vi "SQL模块化.vi"(0 "Database name":string="Test_Database", 1 "Table name":string="Test_Database", 2 "operate option":T1(ring)=enum."Select Data", 3 "primary key (-1)":i32=-1, 4 "Column information":T2[](array[typedef])=[{"column name"="ID", "data type"=enum."Long (I32)", "size"=50, "allow null?"=FALSE}, {"column name"="name", "data type"=enum."String", "size"=50, "allow null?"=TRUE}, {"column name"="number", "data type"=enum."Long (I32)", "size"=50, "allow null?"=TRUE}, {"column name"="date", "data type"=enum."Date/Time", "size"=50, "allow null?"=TRUE}], 5 "Column name":string="ID", 6 "Additional":string, 7 "error in (no error)":errorcluster, 9 "Update Column name":string="name", 10 "Insert Data":string[](array[string])=["5", "D", "5", "2015/1/19 14:41:15"], 11 "Update Data":string="E", 12 "Delete Search Condition":string="ID", 13 "Update Search Condition":string="ID", 14 "Delete Search Condition Value":string="5", 15 "Update Search Condition Value":string="5") -> (8 "columns":string[](array[string])=["ID", "name", "number", "date"], 20 "Data Out":string[][](array[string]), 27 "error out":errorcluster)   [LabVIEW 2017]
uses:
  <vilib>/addons/database/Auxilliary.llb/DB Tools Column Info.ctl
  <vilib>/addons/database/Auxilliary.llb/DB Tools DataTypes.ctl
  <vilib>/addons/database/Auxilliary.llb/DB Tools Transaction.ctl
  <vilib>/addons/database/Connection.llb/DB Tools Open Connec (String).vi
  <vilib>/addons/database/Connection.llb/Conn Transaction.vi
  <vilib>/addons/database/Connection.llb/Conn Execute.vi
  <vilib>/addons/database/Recordset.llb/Rec Fetch Recordset Data (R).vi
  <vilib>/addons/database/Recordset.llb/Rec Destroy - Connection.vi
  <vilib>/addons/database/NI_Database_API.lvlib
panel:
  # "Output"
  # "Input"
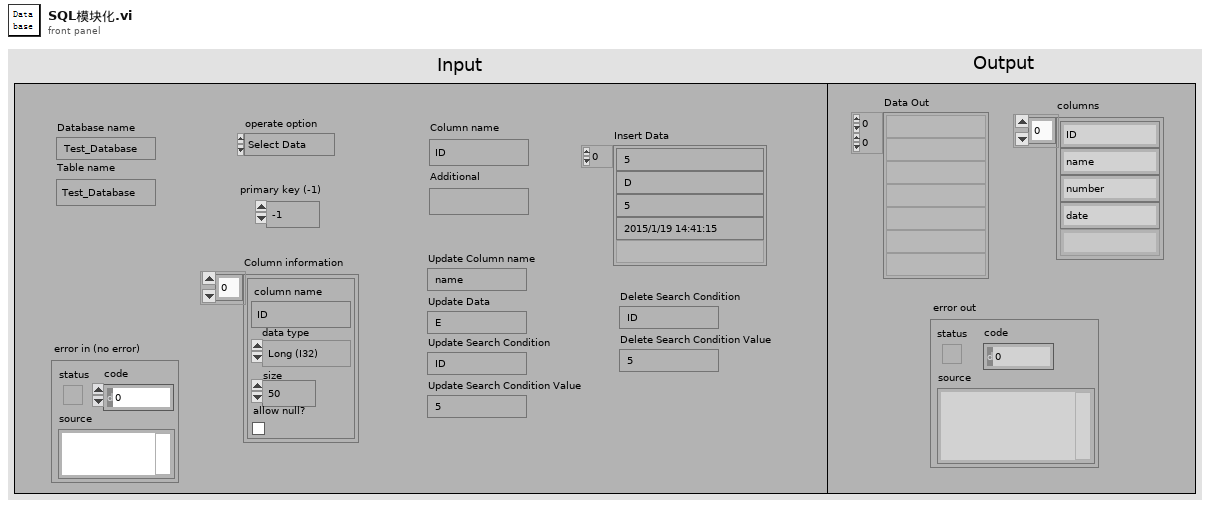
[diagram p1: front panel]
types:
  T1 = enum16{"Create Table", "Select Data", "Insert Data", "Update Data", "Delete Data", "Delete Table", "Select Column"}
  T2 = typedef "NI_Database_API.lvlib/DB Tools Column Info.ctl" = cluster{"column name":string, "data type":T3, "size":i32, "allow null?":bool}
  T3 = typedef "NI_Database_API.lvlib/DB Tools DataTypes.ctl" = enum16{"String", "Long (I32)", "Single (SGL)", "Double (DBL)", "Date/Time", "Binary"}
  T4 = typedef "NI_Database_API.lvlib/Conn ObjectReference.ctl" = refnum<k1>
  T5 = typedef "NI_Database_API.lvlib/DB Tools Transaction.ctl" = enum16{"begin", "commit", "rollback"}
  T6 = typedef "NI_Database_API.lvlib/Rec ObjectReference.ctl" = refnum<k1>
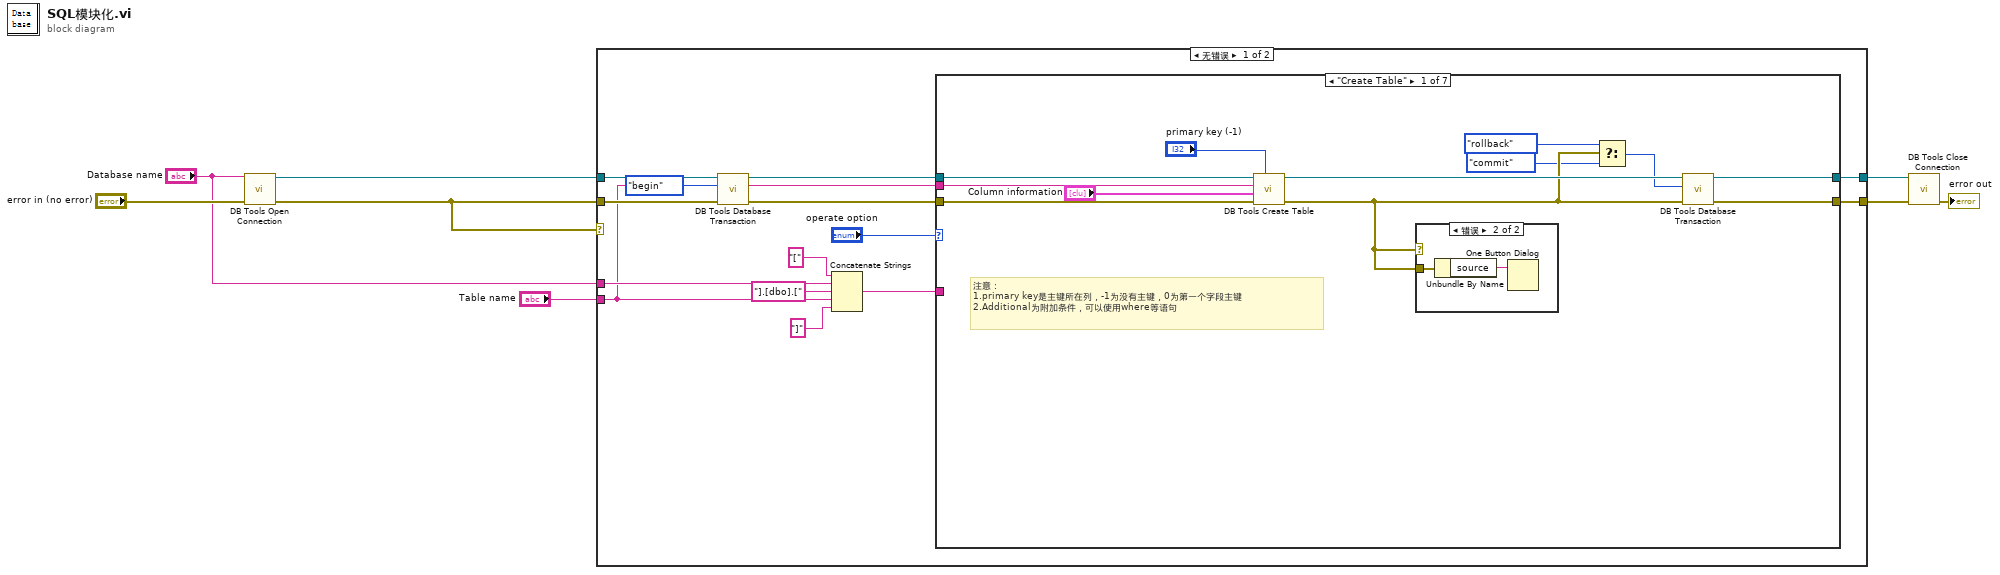
[diagram p0: block diagram]
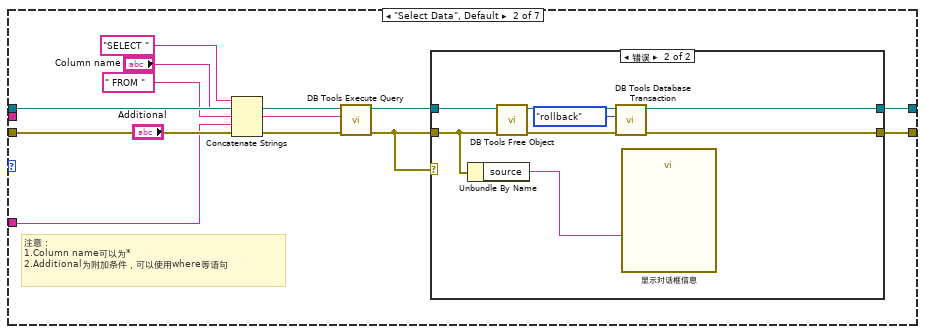
[diagram p3: hidden frame]
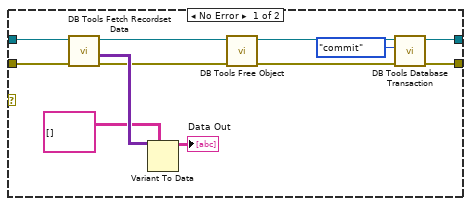
[diagram p4: hidden frame]
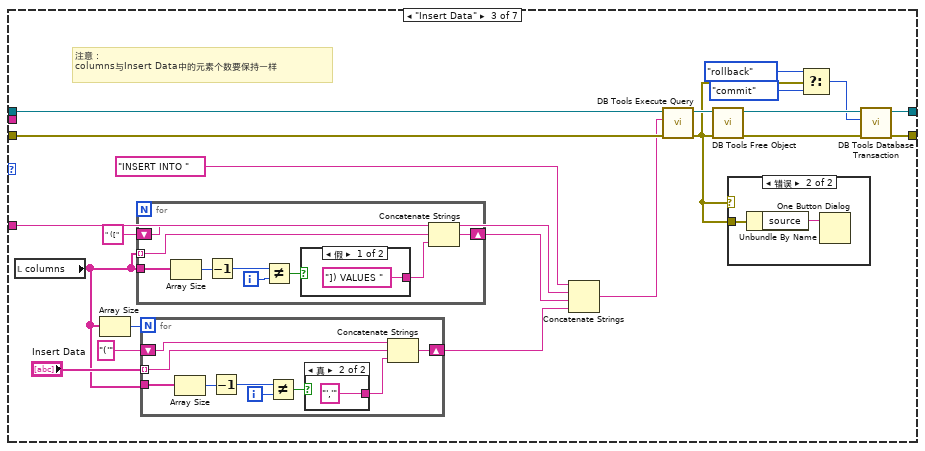
[diagram p5: hidden frame]
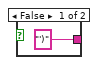
[diagram p7: hidden frame]
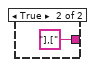
[diagram p8: hidden frame]
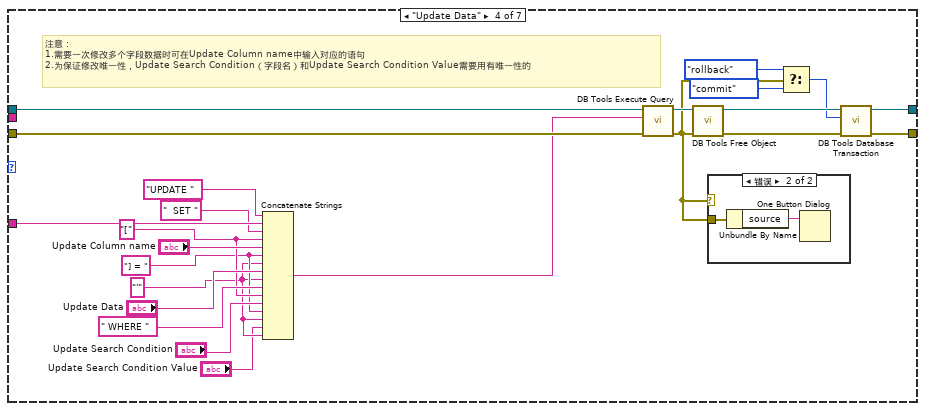
[diagram p9: hidden frame]
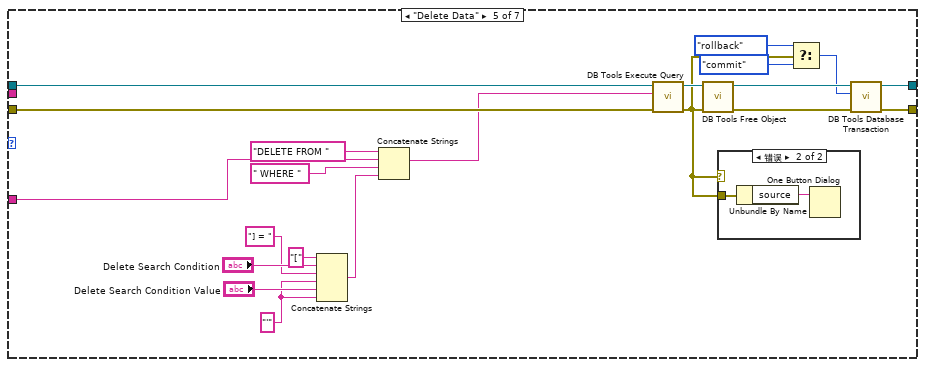
[diagram p11: hidden frame]
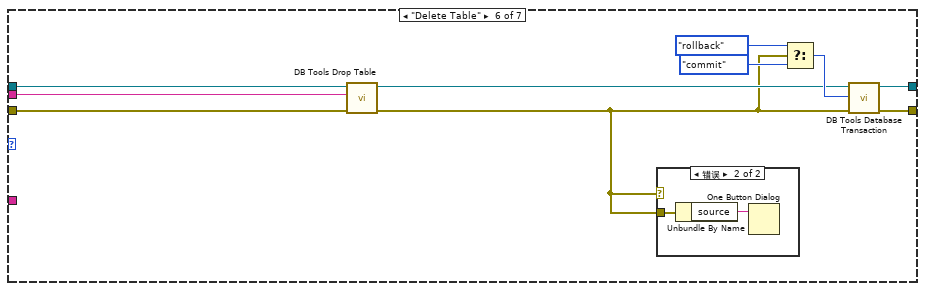
[diagram p13: hidden frame]
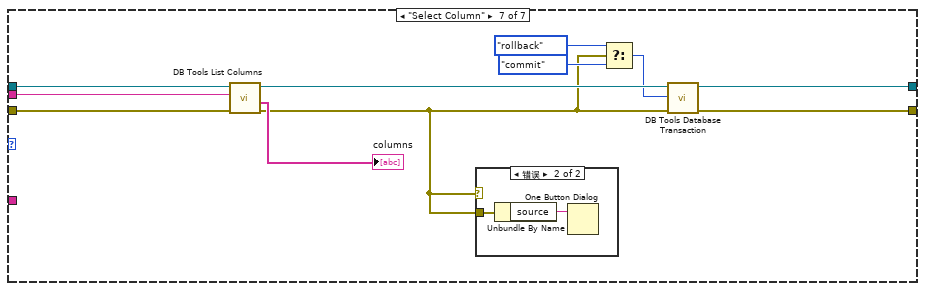
[diagram p15: hidden frame]
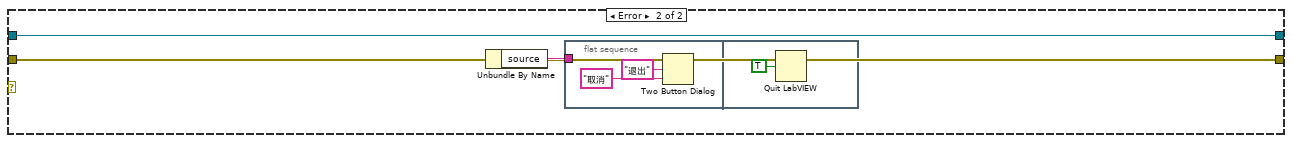
[diagram p17: hidden frame]
diagram:
  n1 = call-poly <vilib>:"DB Tools Open Connection.vi"("error in (no error)"="error in (no error)", "connection information"="Database name") -> ("error out"=w6:errorcluster, "connection reference"=w7:T4)  [unwired: 6 in]
  n2 = case shown="无错误" w6 {
    tunnel: w7 -> [w22 w189]
    tunnel: w6 -> [w21 w187]
    tunnel: [w16 w189] -> w4
    tunnel: [w15 w187] -> w3
    tunnel: "Database name" -> [w10 _]
    tunnel: "Table name" -> [w9 _]
    frame No Error {
      n3 = call-poly <vilib>:"DB Tools Database Transaction.vi"("error in (no error)"=w21, "operation (begin)"=DB_Tools_Transaction."begin", "connection reference"=w22) -> ("error out"=w19:errorcluster, "connection reference out"=w20:T4)  [unwired: 3 in]
      n4 = Concatenate Strings("[", w10, "].[dbo].[", w9, "]") -> (w11:string)
      n5 = case shown="\"Create Table\"" "operate option" {
        tunnel: w20 -> [w33 w48 w88 w127 w150 w171 w184]
        tunnel: w19 -> [w32 w47 w87 w126 w149 w170 w183]
        tunnel: [w30 w46 w80 w129 w152 w165 w179] -> w16
        tunnel: [w24 w45 w79 w128 w151 w164 w178] -> w15
        tunnel: w11 -> [_ w39 w69 w124 w147 _ _]
        tunnel: w9 -> [w31 _ _ _ _ w169 w181]
        frame "Create Table" {
          # "注意：\n1.primary key是主键所在列，-1为没有主键，0为第一个字段主键\n2.Additional为附加条件，可以使用where等语句"
          n6 = call <vilib>:"DB Tools Create Table.vi"("primary key (-1)"="primary key (-1)", "error in (no error)"=w32, "column information"="Column information", "table"=w31, "connection reference"=w33) -> ("error out"=w28:errorcluster, "connection reference out"=w29:T4)  [unwired: 3 in]
          n7 = case shown="错误" w28 {
            tunnel: w28 -> [_ w36]
            frame No Error {
            }
            frame Error {
              n8 = Unbundle By Name(w36) -> ("source"=w35:string)
              n9 = One Button Dialog(message=w35) -> ()  [unwired: 1 in, 1 out]
            }
          }
          n10 = Select(t=DB_Tools_Transaction."rollback" ("operation (begin)"), s=w28, f=DB_Tools_Transaction."commit" ("operation (begin)")) -> (s? t:f=w25:T5)
          n11 = call-poly <vilib>:"DB Tools Database Transaction.vi"("error in (no error)"=w28, "operation (begin)"=w25, "connection reference"=w29) -> ("error out"=w24:errorcluster, "connection reference out"=w30:T4)  [unwired: 3 in]
        }
        frame "Select Data", Default {
          # "注意：\n1.Column name可以为*\n2.Additional为附加条件，可以使用where等语句"
          n12 = Concatenate Strings("SELECT ", "Column name", " FROM ", w39, "Additional") -> (w41:string)
          n13 = call-poly <vilib>:"DB Tools Execute Query.vi"("error in (no error)"=w47, "SQL query"=w41, "connection reference"=w48) -> ("error out"=w37:errorcluster, "recordset reference"=w38:T6)  [unwired: 5 in]
          n14 = case shown="错误" w37 {
            tunnel: [w54 w65] -> w46
            tunnel: [w53 w64] -> w45
            tunnel: w38 -> [w60 w68]
            tunnel: w37 -> [w57 w62]
            frame No Error {
              n15 = call-poly <vilib>:"DB Tools Fetch Recordset Data.vi"("error in (no error)"=w57, "recordset reference"=w60) -> ("error out"=w49:errorcluster, "recordset data"=w59:variant[][], "recordset reference out"=w50:T6)  [unwired: 3 in]
              n16 = Variant To Data(type=string[][] [], Variant=w59) -> (data=→"Data Out":string[][])  [unwired: 1 in, 1 out]
              n17 = call-poly <vilib>:"DB Tools Free Object.vi"("error in (no error)"=w49, "recordset reference"=w50) -> ("error out"=w55:errorcluster, "connection reference"=w56:T4)  [unwired: 8 in]
              n18 = call-poly <vilib>:"DB Tools Database Transaction.vi"("error in (no error)"=w55, "operation (begin)"=DB_Tools_Transaction."commit", "connection reference"=w56) -> ("error out"=w53:errorcluster, "connection reference out"=w54:T4)  [unwired: 3 in]
            }
            frame Error {
              n19 = Unbundle By Name(w62) -> ("source"=w61:string)
              n20 = call-poly <vilib>:"DB Tools Free Object.vi"("error in (no error)"=w62, "recordset reference"=w68) -> ("error out"=w66:errorcluster, "connection reference"=w67:T4)  [unwired: 8 in]
              n21 = call-poly <vilib>:"DB Tools Database Transaction.vi"("error in (no error)"=w66, "operation (begin)"=DB_Tools_Transaction."rollback", "connection reference"=w67) -> ("error out"=w64:errorcluster, "connection reference out"=w65:T4)  [unwired: 3 in]
              n22 = call "显示对话框信息"("Message"=w61) -> ()  [unwired: 9 in, 2 out]
            }
          }
        }
        frame "Insert Data" {
          # "注意：\ncolumns与Insert Data中的元素个数要保持一样"
          n23 = local read "columns"() -> (w75:string[])
          n24 = Array Size(array=w75) -> (size(s)=w76:i32)
          n25 = for {
            tunnel: w75 -> [w111] mode=indexing
            shift-right: [w110] -> w83
            shift-left: " ([" -> [w109]
            tunnel: w75 -> [w107]
            i -> [w104]
            n26 = Array Size(array=w107) -> (size(s)=w106:i32)
            n27 = Decrement(x=w106) -> (x-1=w105:i32)
            n28 = Not Equal?(x=w105, y=w104) -> (x != y?=w103:bool)
            n29 = case shown="假" w103 {
              tunnel: ["]) VALUES " ("字符串") "],[" ("字符串")] -> w108
              frame False {
              }
              frame True {
              }
            }
            n30 = Concatenate Strings(w109, w111, w108) -> (w110:string)
          }
          n31 = for {
            N: w76 -> [_]
            tunnel: "Insert Data" -> [w100] mode=indexing
            shift-right: [w99] -> w82
            shift-left: "('" -> [w98]
            tunnel: w75 -> [w96]
            i -> [w93]
            n32 = Array Size(array=w96) -> (size(s)=w95:i32)
            n33 = Decrement(x=w95) -> (x-1=w94:i32)
            n34 = Not Equal?(x=w94, y=w93) -> (x != y?=w92:bool)
            n35 = case shown="真" w92 {
              tunnel: ["')" ("字符串") "','" ("字符串")] -> w97
              frame False {
              }
              frame True {
              }
            }
            n36 = Concatenate Strings(w98, w100, w97) -> (w99:string)
          }
          n37 = Concatenate Strings("INSERT INTO ", w69, w83, w82) -> (w81:string)
          n38 = call-poly <vilib>:"DB Tools Execute Query.vi"("error in (no error)"=w87, "SQL query"=w81, "connection reference"=w88) -> ("error out"=w74:errorcluster, "recordset reference"=w89:T6)  [unwired: 5 in]
          n39 = call-poly <vilib>:"DB Tools Free Object.vi"("error in (no error)"=w74, "recordset reference"=w89) -> ("error out"=w77:errorcluster, "connection reference"=w78:T4)  [unwired: 8 in]
          n40 = case shown="错误" w74 {
            tunnel: w74 -> [_ w91]
            frame No Error {
            }
            frame Error {
              n41 = Unbundle By Name(w91) -> ("source"=w90:string)
              n42 = One Button Dialog(message=w90) -> ()  [unwired: 1 in, 1 out]
            }
          }
          n43 = Select(t=DB_Tools_Transaction."rollback" ("operation (begin)"), s=w74, f=DB_Tools_Transaction."commit" ("operation (begin)")) -> (s? t:f=w71:T5)
          n44 = call-poly <vilib>:"DB Tools Database Transaction.vi"("error in (no error)"=w77, "operation (begin)"=w71, "connection reference"=w78) -> ("error out"=w79:errorcluster, "connection reference out"=w80:T4)  [unwired: 3 in]
        }
        frame "Update Data" {
          w116 = "'"
          w117 = "] = "
          w118 = "["
          # "注意：\n1.需要一次修改多个字段数据时可在Update Column name中输入对应的语句\n2.为保证修改唯一性，Update Search Condition（字段名）和Update Search Condition Value需要用有唯一性的"
          n45 = Concatenate Strings("UPDATE ", w124, "  SET ", w118, "Update Column name", w117, w116, "Update Data", w116, " WHERE ", w118, "Update Search Condition", w117, w116, "Update Search Condition Value", w116) -> (w114:string)
          n46 = call-poly <vilib>:"DB Tools Execute Query.vi"("error in (no error)"=w126, "SQL query"=w114, "connection reference"=w127) -> ("error out"=w133:errorcluster, "recordset reference"=w136:T6)  [unwired: 5 in]
          n47 = call-poly <vilib>:"DB Tools Free Object.vi"("error in (no error)"=w133, "recordset reference"=w136) -> ("error out"=w134:errorcluster, "connection reference"=w135:T4)  [unwired: 8 in]
          n48 = case shown="错误" w133 {
            tunnel: w133 -> [_ w138]
            frame No Error {
            }
            frame Error {
              n49 = Unbundle By Name(w138) -> ("source"=w137:string)
              n50 = One Button Dialog(message=w137) -> ()  [unwired: 1 in, 1 out]
            }
          }
          n51 = Select(t=DB_Tools_Transaction."rollback" ("operation (begin)"), s=w133, f=DB_Tools_Transaction."commit" ("operation (begin)")) -> (s? t:f=w130:T5)
          n52 = call-poly <vilib>:"DB Tools Database Transaction.vi"("error in (no error)"=w134, "operation (begin)"=w130, "connection reference"=w135) -> ("error out"=w128:errorcluster, "connection reference out"=w129:T4)  [unwired: 3 in]
        }
        frame "Delete Data" {
          w141 = "'"
          n53 = Concatenate Strings("[", "Delete Search Condition", "] = ", w141, "Delete Search Condition Value", w141) -> (w140:string)
          n54 = Concatenate Strings("DELETE FROM ", w147, " WHERE ", w140) -> (w139:string)
          n55 = call-poly <vilib>:"DB Tools Execute Query.vi"("error in (no error)"=w149, "SQL query"=w139, "connection reference"=w150) -> ("error out"=w156:errorcluster, "recordset reference"=w159:T6)  [unwired: 5 in]
          n56 = call-poly <vilib>:"DB Tools Free Object.vi"("error in (no error)"=w156, "recordset reference"=w159) -> ("error out"=w157:errorcluster, "connection reference"=w158:T4)  [unwired: 8 in]
          n57 = case shown="错误" w156 {
            tunnel: w156 -> [_ w161]
            frame No Error {
            }
            frame Error {
              n58 = Unbundle By Name(w161) -> ("source"=w160:string)
              n59 = One Button Dialog(message=w160) -> ()  [unwired: 1 in, 1 out]
            }
          }
          n60 = Select(t=DB_Tools_Transaction."rollback" ("operation (begin)"), s=w156, f=DB_Tools_Transaction."commit" ("operation (begin)")) -> (s? t:f=w153:T5)
          n61 = call-poly <vilib>:"DB Tools Database Transaction.vi"("error in (no error)"=w157, "operation (begin)"=w153, "connection reference"=w158) -> ("error out"=w151:errorcluster, "connection reference out"=w152:T4)  [unwired: 3 in]
        }
        frame "Delete Table" {
          n62 = call <vilib>:"DB Tools Drop Table.vi"("error in (no error)"=w170, "table"=w169, "connection reference"=w171) -> ("error out"=w162:errorcluster, "connection reference out"=w163:T4)  [unwired: 5 in]
          n63 = case shown="错误" w162 {
            tunnel: w162 -> [_ w173]
            frame No Error {
            }
            frame Error {
              n64 = Unbundle By Name(w173) -> ("source"=w172:string)
              n65 = One Button Dialog(message=w172) -> ()  [unwired: 1 in, 1 out]
            }
          }
          n66 = Select(t=DB_Tools_Transaction."rollback" ("operation (begin)"), s=w162, f=DB_Tools_Transaction."commit" ("operation (begin)")) -> (s? t:f=w166:T5)
          n67 = call-poly <vilib>:"DB Tools Database Transaction.vi"("error in (no error)"=w162, "operation (begin)"=w166, "connection reference"=w163) -> ("error out"=w164:errorcluster, "connection reference out"=w165:T4)  [unwired: 3 in]
        }
        frame "Select Column" {
          n68 = call <vilib>:"DB Tools List Columns.vi"("error in (no error)"=w183, "table"=w181, "connection reference"=w184) -> ("error out"=w175:errorcluster, "columns"=→"columns":string[], "connection reference out"=w180:T4)  [unwired: 1 in, 1 out]
          n69 = case shown="错误" w175 {
            tunnel: w175 -> [_ w186]
            frame No Error {
            }
            frame Error {
              n70 = Unbundle By Name(w186) -> ("source"=w185:string)
              n71 = One Button Dialog(message=w185) -> ()  [unwired: 1 in, 1 out]
            }
          }
          n72 = Select(t=DB_Tools_Transaction."rollback" ("operation (begin)"), s=w175, f=DB_Tools_Transaction."commit" ("operation (begin)")) -> (s? t:f=w174:T5)
          n73 = call-poly <vilib>:"DB Tools Database Transaction.vi"("error in (no error)"=w175, "operation (begin)"=w174, "connection reference"=w180) -> ("error out"=w178:errorcluster, "connection reference out"=w179:T4)  [unwired: 3 in]
        }
      }
    }
    frame Error {
      n74 = Unbundle By Name(w187) -> ("source"=w188:string)
      n75 = flat-sequence {
        tunnel: w188 -> [w192]
        frame #0 {
          n76 = Two Button Dialog(message=w192, 1:"取消" ("T按钮名称（“确定”）"), 2:"退出" ("T按钮名称（“确定”）")) -> ()  [unwired: 1 out]
        }
        frame #1 {
          n77 = Quit LabVIEW(quit? (T)=TRUE ("退出？(T)")) -> ()
        }
      }
    }
  }
  n78 = call <vilib>:"DB Tools Close Connection.vi"("error in (no error)"=w3, "connection reference"=w4) -> ("error out"=→"error out":errorcluster)  [unwired: 5 in]
